vi "Number Of World The.vi"() -> ()   [LabVIEW 2019]
panel:
  out "Numeric":i16
  in  "String":string
  # "shuchu the de ge shu"
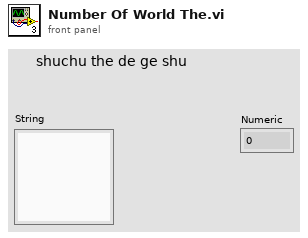
[diagram p1: front panel]
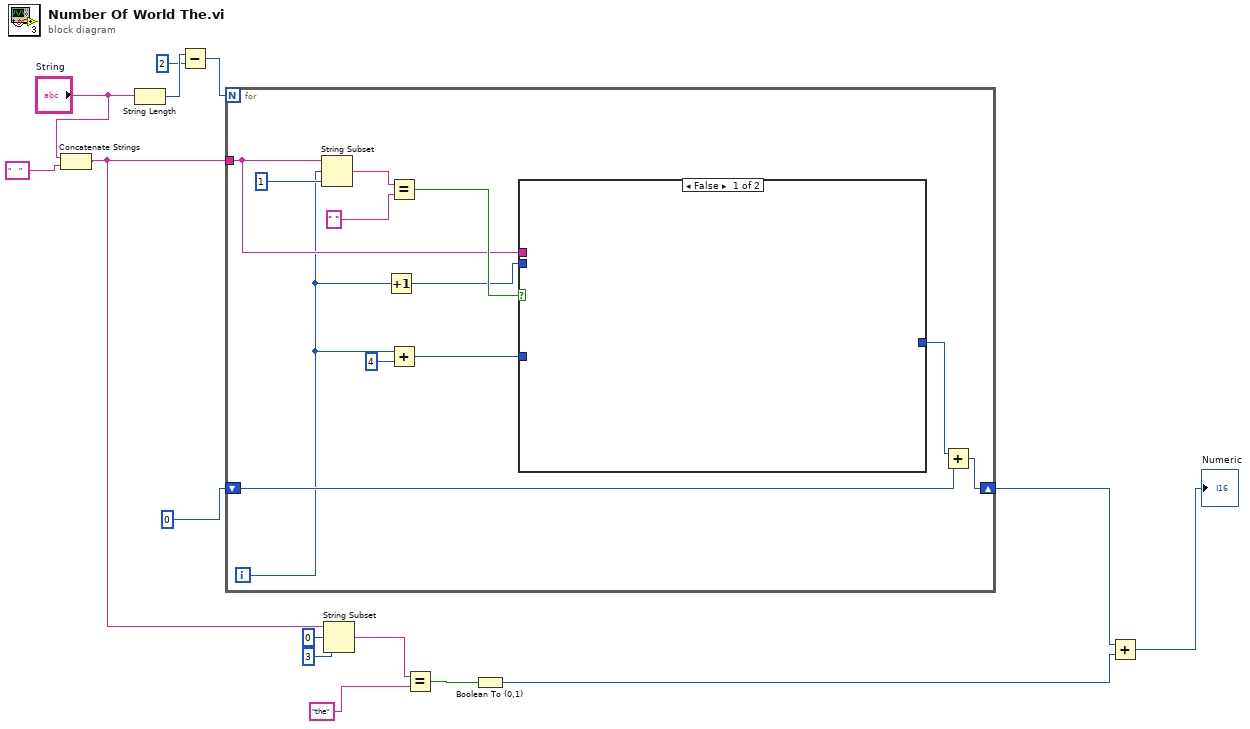
[diagram p0: block diagram]
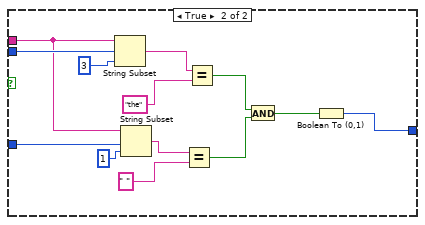
[diagram p2: hidden frame]
diagram:
  n1 = Concatenate Strings("String", "    ") -> (w3:string)
  n2 = String Length(string="String") -> (length=w14:i32)
  n3 = Subtract(x=w14, y=2) -> (x-y=w15:i32)
  n4 = for {
    N: w15 -> [_]
    tunnel: w3 -> [w25]
    shift-right: [w17] -> w6
    shift-left: 0 -> [w24]
    i -> [w20]
    n5 = String Subset(string=w25, offset (0)=w20, length (rest)=1 ("length (rest)")) -> (substring=w23:string)
    n6 = Increment(x=w20) -> (x+1=w21:i32)
    n7 = Equal?(x=w23, y=" ") -> (x = y?=w26:bool)
    n8 = Add(x=w20, y=4) -> (x+y=w18:i32)
    n9 = case shown="False" w26 {
      tunnel: w25 -> [_ w34]
      tunnel: w21 -> [_ w40]
      tunnel: w18 -> [_ w36]
      tunnel: [_ w28] -> w16
      frame False {
      }
      frame True {
        n10 = String Subset(string=w34, offset (0)=w40, length (rest)=3 ("length (rest)")) -> (substring=w38:string)
        n11 = String Subset(string=w34, offset (0)=w36, length (rest)=1 ("length (rest)")) -> (substring=w33:string)
        n12 = Equal?(x=w33, y=" ") -> (x = y?=w30:bool)
        n13 = Equal?(x=w38, y="the") -> (x = y?=w31:bool)
        n14 = And(x=w31, y=w30) -> (x .and. y?=w29:bool)
        n15 = Boolean To (0,1)(Boolean=w29) -> (0, 1=w28:i16)
      }
    }
    n16 = Add(x=w16, y=w24) -> (x+y=w17:i32)
  }
  n17 = String Subset(string=w3, offset (0)=0, length (rest)=3 ("length (rest)")) -> (substring=w8:string)
  n18 = Equal?(x=w8, y="the") -> (x = y?=w7:bool)
  n19 = Boolean To (0,1)(Boolean=w7) -> (0, 1=w4:i16)
  n20 = Add(x=w6, y=w4) -> (x+y=→"Numeric":i32)
